vi "Initialize.vi"(8 "error in (no error)":errorcluster, 10 "Fluidics Configuration":T1={"Serial Port"="COM3", "Device Type"=enum."Disabled"}) -> (0 "error out":errorcluster, 3 "Autosampler out":refnum<class "Autosampler.lvclass">)   [LabVIEW 2023, in "Autosampler.lvlib" / "Autosampler.lvclass"]
uses:
  Autosampler.lvclass
  Resources/Type Defs/Autosampler Configuration.ctl
  Autosampler.lvclass/Autosampler.ctl
panel:
  in  "Autosampler in":refnum<class "Autosampler.lvclass">
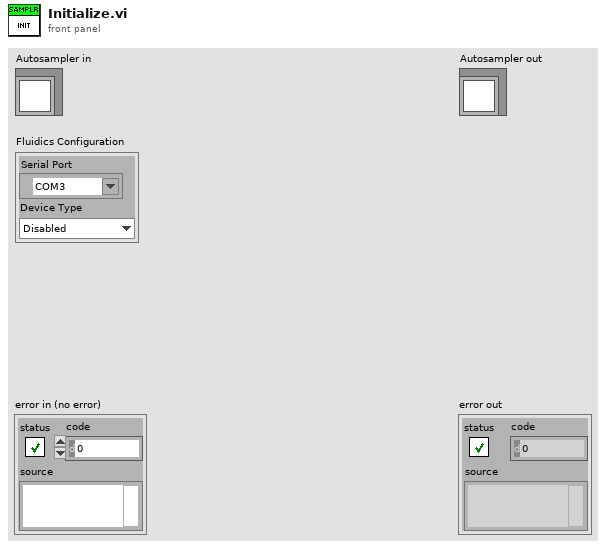
[diagram p1: front panel]
types:
  T1 = typedef "Autosampler Configuration.ctl" = cluster{"Serial Port":refnum<visa-resource-name>, "Device Type":enum16{"Disabled", "Simulate", "Alltesta"}}
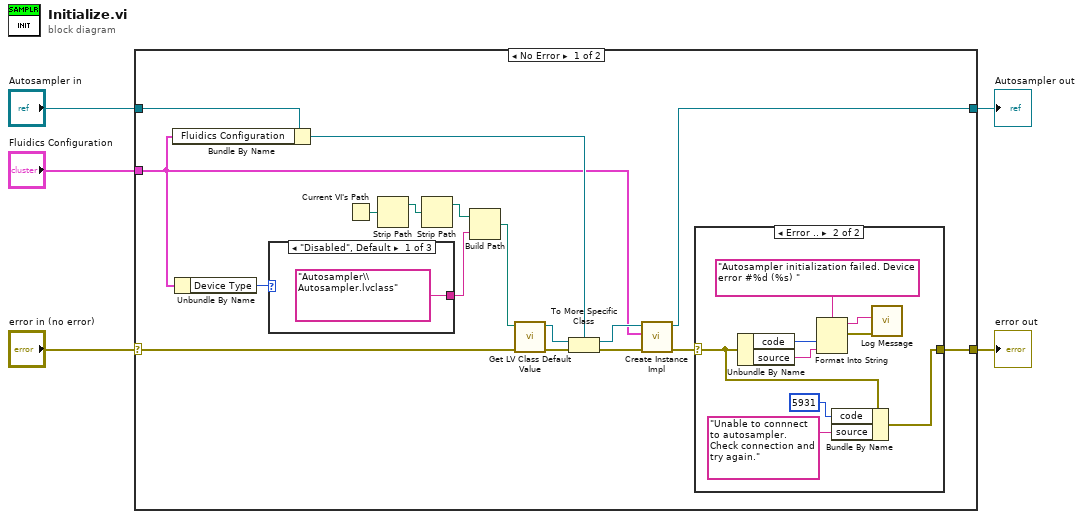
[diagram p0: block diagram]
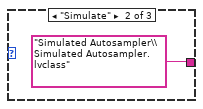
[diagram p3: hidden frame]
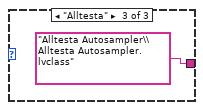
[diagram p4: hidden frame]
diagram:
  n1 = case shown="No Error" "error in (no error)" {
    selector: "error in (no error)" -> [w16 w37]
    tunnel: [w6 w37] -> w4
    tunnel: [w8 w36] -> w2
    tunnel: "Autosampler in" -> [w11 w36]
    tunnel: "Fluidics Configuration" -> [w9 _]
    frame No Error {
      n2 = Bundle By Name(cluster=w11, "Fluidics Configuration"=w9) -> (w10:refnum<class "Autosampler.lvclass">)
      n3 = Unbundle By Name(w9) -> ("Device Type"=w12:enum16{"Disabled", "Simulate", "Alltesta"})
      n4 = case shown="\"Disabled\", Default" w12 {
        tunnel: ["Autosampler\\Autosampler.lvclass" "Simulated Autosampler\\Simulated Autosampler.lvclass" "Alltesta Autosampler\\Alltesta Autosampler.lvclass"] -> w22
        frame "Disabled", Default {
        }
        frame "Simulate" {
        }
        frame "Alltesta" {
        }
      }
      n5 = Current VI's Path() -> (path=w19:path)
      n6 = Strip Path(path=w19) -> (stripped path=w20:path)  [unwired: 1 out]
      n7 = Strip Path(path=w20) -> (stripped path=w21:path)  [unwired: 1 out]
      n8 = Build Path(base path=w21, name or relative path=w22) -> (appended path=w15:path)
      n9 = call <vilib>:"Get LV Class Default Value.vi"("error in (no error)"=w16, "class path"=w15) -> ("error out"=w18:errorcluster, "object"=w14:refnum<class>)  [unwired: 8 in]
      n10 = To More Specific Class(target class=w10, reference=w14, error in=w18) -> (specific class reference=w13:refnum<class "Autosampler.lvclass">, error out=w17:errorcluster)
      n11 = call-dynamic "Create Instance Impl.vi"("error in (no error)"=w17, "Fluidics Configuration"=w9, "Autosampler in"=w13) -> ("error out"=w7:errorcluster, "Autosampler out"=w8:refnum<class "Autosampler.lvclass">)  [unwired: 7 in]
      n12 = case shown="Error .." w7 {
        selector: w7 -> [w23 w28]
        tunnel: [w23 w27] -> w6
        frame No Error {
        }
        frame Error {
          n13 = Unbundle By Name(w28) -> ("code"=w29:i32, "source"=w24:string)
          n14 = Format Into String(format string="Autosampler initialization failed. Device error #%d (%s) ", w29, w24) -> (resulting string=w31:string, error out=w30:errorcluster)  [unwired: 2 in]
          n15 = Bundle By Name(cluster=w28, "code"=5931 ("Autosampler connection error"), "source"="Unable to connnect to autosampler. Check connection and try again.") -> (w27:errorcluster)
          n16 = call "Log Message.vi"("error constant"=w30, "input"=w31) -> ()  [unwired: 8 in, 2 out]
        }
      }
    }
    frame Error {
    }
  }
  "error out" <- w4
  "Autosampler out" <- w2
